vi "Build Path Test.vi"(8 "error in":errorcluster, 11 "Report Generator in":refnum<class "Report Generator.lvclass">) -> (0 "error out":errorcluster, 3 "Report Generator out":refnum<class "Report Generator.lvclass">)   [LabVIEW 2018, in "Report Generator.lvlib" / "Report Generator.lvclass"]
uses:
  Report Generator.lvclass
  Report Generator.lvclass/Report Generator.ctl
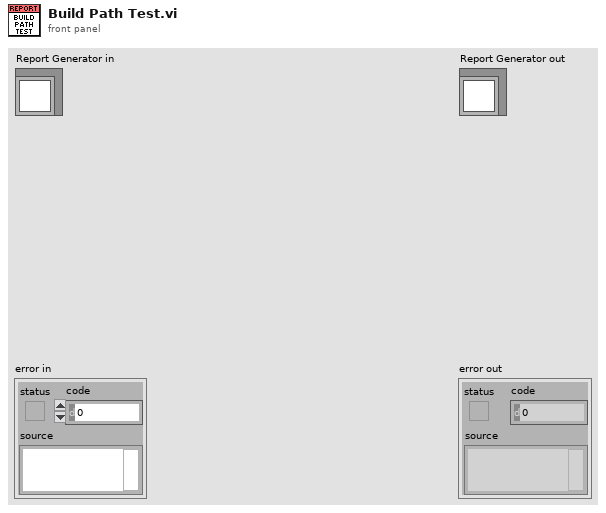
[diagram p1: front panel]
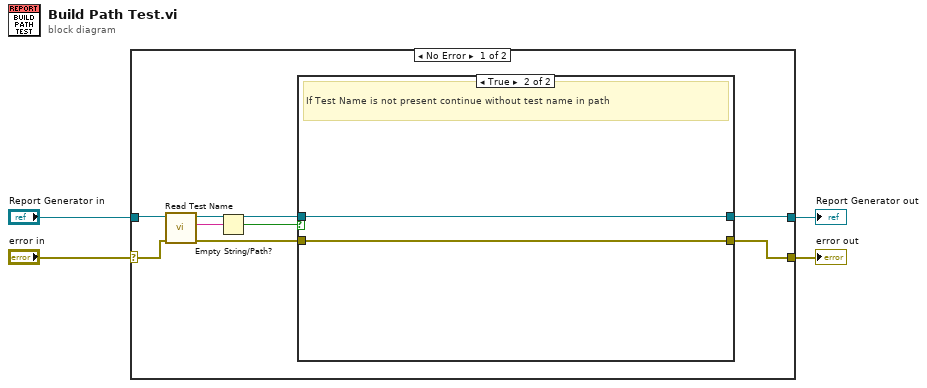
[diagram p0: block diagram]
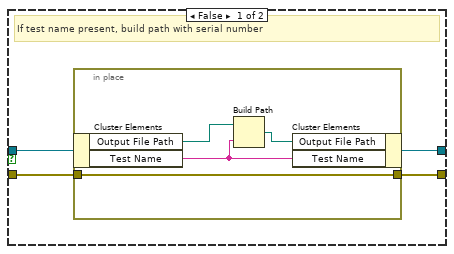
[diagram p2: hidden frame]
diagram:
  n1 = case shown="No Error" "error in" {
    selector: "error in" -> [w5 w24]
    tunnel: [w10 w24] -> w3
    tunnel: [w11 w23] -> w1
    tunnel: "Report Generator in" -> [w9 w23]
    frame No Error {
      n2 = call "Read Test Name.vi"("error in (no error)"=w5, "Report Generator in"=w9) -> ("error out"=w6:errorcluster, "Test Name"=w7:string, "Report Generator out"=w8:refnum<class "Report Generator.lvclass">)  [unwired: 7 in]
      n3 = Empty String/Path?(string/path=w7) -> (empty?=w12:bool)
      n4 = case shown="True" w12 {
        tunnel: w8 -> [w16 w22]
        tunnel: w6 -> [w14 w21]
        tunnel: [w15 w22] -> w11
        tunnel: [w13 w21] -> w10
        frame False {
          # "If test name present, build path with serial number"
          n5 = in-place {
            in-place-border: w14 -> [w17]
            in-place-border: [w17] -> w13
            n6 = in-place-cluster #1(w16) -> ("Output File Path"=w20:path, "Test Name"=w19:string)
            n7 = Build Path(base path=w20, name or relative path=w19) -> (appended path=w18:path)
            n8 = in-place-cluster #1("Output File Path"=w18, "Test Name"=w19) -> (w15:refnum<class "Report Generator.lvclass">)
          }
        }
        frame True {
          # "If Test Name is not present continue without test name in path"
        }
      }
    }
    frame Error {
    }
  }
  "error out" <- w3
  "Report Generator out" <- w1
